vi "Write Model Startup View.vi"(10 "Startup View":refnum<class "IViewable.lvclass">, 11 "IModel In":refnum<class "IModel.lvclass">) -> (3 "IModel Out":refnum<class "IModel.lvclass">)   [LabVIEW 2015, in "IModel.lvlib" / "IModel.lvclass"]
uses:
  IModel.lvclass
  IViewable/IViewable/IViewable.lvclass
  IViewManager/IViewManager Messages/Launch Nested Views Msg/Launch Nested Views Msg.lvclass/Launch Nested Views Msg.ctl
  IViewManager/IViewManager/IViewManager.lvclass/IViewManager.ctl
  IViewManager/IViewManager Messages/Launch Nested Views Msg/Launch Nested Views Msg.lvclass
  IViewManager/IViewManager/IViewManager.lvclass
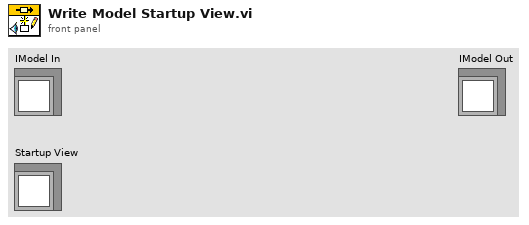
[diagram p1: front panel]
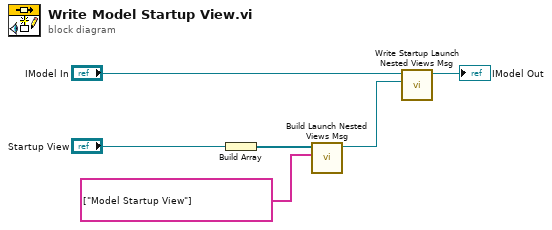
[diagram p0: block diagram]
diagram:
  n1 = Build Array("Startup View") -> (w4:refnum<class "IViewable.lvclass">[])
  n2 = call "Build Launch Nested Views Msg.vi"("View Labels"=string[] ["Model Startup View"] ("View Labels (optional)"), "Nested Views"=w4) -> ("Launch Nested Views Msg out"=w2:refnum<class "Launch Nested Views Msg.lvclass">)  [unwired: 8 in, 1 out]
  n3 = call "Write Startup Launch Nested Views Msg.vi"("Launch Nested Views Msg"=w2, "IViewManager in"="IModel In") -> ("IViewManager out"=→"IModel Out":refnum<class "IModel.lvclass">)  [unwired: 8 in, 1 out]
